vi "RampToSet.vi"(8 "error in (no error)":errorcluster, 11 "Instrument.VRM in":refnum<class "Instrument.OxfordVRM.lvclass">) -> (0 "error out":errorcluster, 2 "Response":string, 3 "Instrument.VRM out":refnum<class "Instrument.OxfordVRM.lvclass">)   [LabVIEW 2019, in "Instrument.OxfordVRM.lvclass"]
uses:
  Instrument.OxfordVRM.lvclass
  Typedefs/Instrument.VRM.protectedCommands-enum.ctl
  1b310fa8-6495-4ebe-9d13-ec9611e0ed8a.vi
  1b310fa8-6495-4ebe-9d13-ec9611e0ed8a.vi/89bbbbc0-76c2-439c-85b9-13f9782c8812.vi
  1b310fa8-6495-4ebe-9d13-ec9611e0ed8a.vi/d6a14854-4f97-4a59-9534-d90670edf1af.vi
  <vilib>/Utility/Data Type/Get Type Information.vi
  <vilib>/JDP Science/JSONtext/JSON text to Variant.vi
  <vilib>/JDP Science/JSONtext/LVClass Serializer/JSONtext LVClass Serializer.lvclass
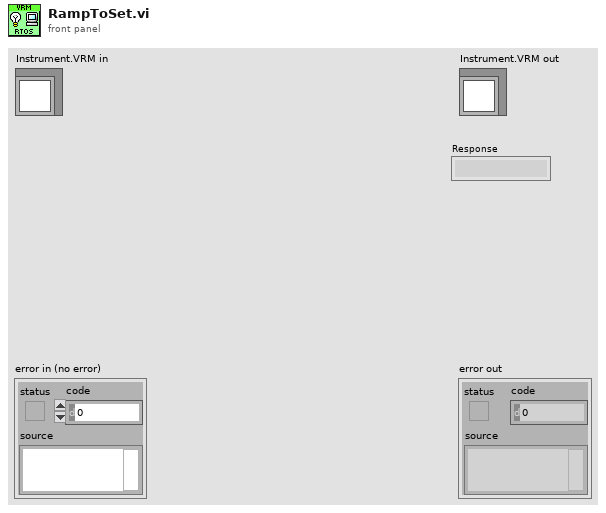
[diagram p1: front panel]
types:
  T1 = typedef "Instrument.OxfordVRM.lvclass/Instrument.VRM.protectedCommands-enum.ctl" = enum16{"Hold", "RampToSet", "RampToZero", "Clamp", "SetTarget", "GetStatus", "GetTarget", "GetField"}
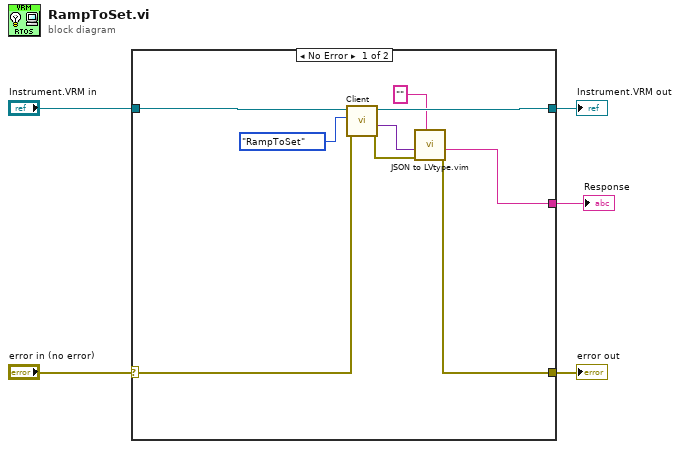
[diagram p0: block diagram]
diagram:
  n1 = case shown="No Error" "error in (no error)" {
    selector: "error in (no error)" -> [w13 w16]
    tunnel: [w10 w16] -> w4
    tunnel: [w12 w15] -> w2
    tunnel: "Instrument.VRM in" -> [w14 w15]
    tunnel: [w11 _] -> w1
    frame No Error {
      n2 = call-dynamic "Client.vi"("error in (no error)"=w13, "Command in"=Instrument.VRM.protectedCommands-enum."RampToSet" ("protectedCommands"), "Instrument in"=w14) -> ("error out"=w6:errorcluster, "Data out"=w8:variant, "Instrument out"=w12:refnum<class "Instrument.OxfordVRM.lvclass">)  [unwired: 5 in, 1 out]
      n3 = call "JSON to LVtype.vim"("type"="", "error in (no error)"=w6, "JSON Data in"=w8) -> ("error out"=w10:errorcluster, "Data out"=w11:string)  [unwired: 7 in]
    }
    frame Error {
    }
  }
  "error out" <- w4
  "Instrument.VRM out" <- w2
  "Response" <- w1
